vi "TB-Init History.vi"(0 "state":T1, 5 "Num Buffers":i32, 7 "XYGraph in":refnum<vi>) -> (4 "history":cluster{dbl[], dbl[]}[](array[cluster]))   [LabVIEW 2020]
uses:
  Typedefs/TB-Runtime state.ctl
  <vilib>/sound2/lvsound2.llb/Sound File Refnum.ctl
  Typedefs/TB-Setup Log.ctl
  Typedefs/TB-Analysis State.ctl
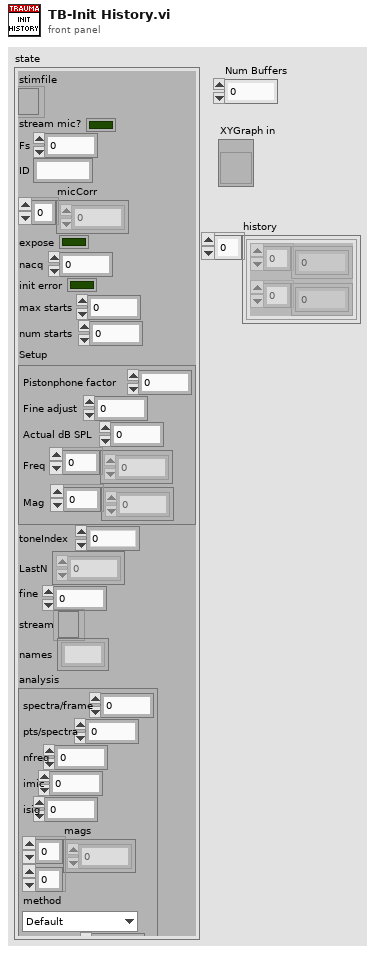
[diagram p1: front panel]
types:
  T1 = typedef "TB-Runtime state.ctl" = cluster{"stimfile":T2, "stream mic?":bool, "Fs":dbl, "ID":string, "micCorr":dbl[], "expose":bool, "nacq":i32, "init error":bool, "max starts":i32, "num starts":i32, "Setup":T3, "toneIndex":i32, "LastN":dbl[], "fine":dbl, "stream":refnum<file>, "names":string[], "analysis":T4}
  T2 = typedef "Sound File Refnum.ctl" = refnum<file>
  T3 = typedef "TB-Setup Log.ctl" = cluster{"Pistonphone factor":dbl, "Fine adjust":dbl, "Actual dB SPL":dbl, "Freq":dbl[], "Mag":dbl[]}
  T4 = typedef "TB-Analysis State.ctl" = cluster{"spectra/frame":i32, "pts/spectra":i32, "nfreq":i32, "imic":i32, "isig":i32, "mags":dbl[][], "method":enum16{"Default", "Periodogram", "Cross-spectrum"}, "cspd scale":dbl}
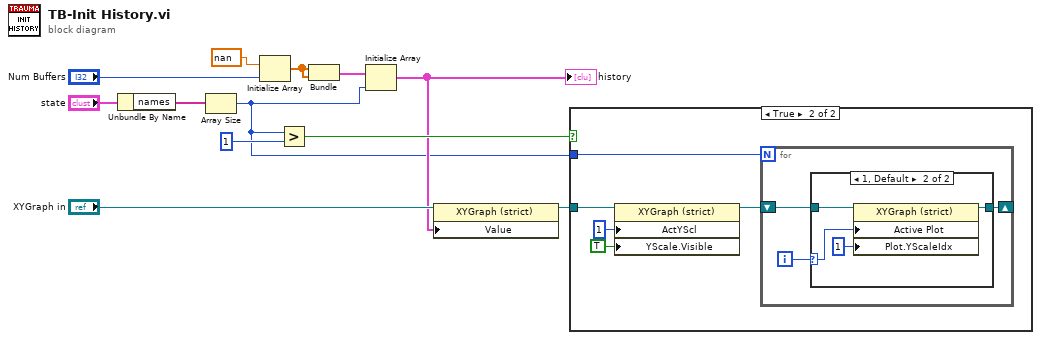
[diagram p0: block diagram]
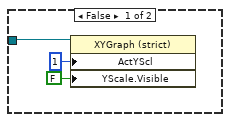
[diagram p2: hidden frame]
diagram:
  n1 = Unbundle By Name("state") -> ("names"=w11:string[])
  n2 = Array Size(array=w11) -> (size(s)=w1:i32)
  n3 = Initialize Array(nan ("element"), "Num Buffers") -> (w9:dbl[])
  n4 = Greater?(x=w1, y=1) -> (0:w6:bool)
  n5 = Bundle(w9, w9) -> (w8:cluster{dbl[], dbl[]})  [unwired: 1 in]
  n6 = Initialize Array(w8, w1) -> (w3:cluster{dbl[], dbl[]}[])
  "history" <- w3
  n7 = property class="XYGraph (strict)"(reference="XYGraph in", "Value"=w3) -> (reference out=w5:refnum<vi>)  [unwired: 1 in, 1 out]
  n8 = case shown="True" w6 {
    tunnel: w5 -> [w15 w18]
    tunnel: w1 -> [_ w16]
    frame False {
      n9 = property class="XYGraph (strict)"(reference=w15, "ActYScl"=1 ("Active Y Scale"), "YScale.Visible"=FALSE ("Y Scale.Visible")) -> ()  [unwired: 1 in, 2 out]
    }
    frame True {
      n10 = property class="XYGraph (strict)"(reference=w18, "ActYScl"=1 ("Active Y Scale"), "YScale.Visible"=TRUE ("Y Scale.Visible")) -> (reference out=w17:refnum<vi>)  [unwired: 1 in, 1 out]
      n11 = for {
        N: w16 -> [_]
        shift-right: [w22] -> _
        shift-left: w17 -> [w23]
        i -> [w21]
        n12 = case shown="1, Default" w21 {
          selector: w21 -> [_ w26]
          tunnel: w23 -> [w24 w28]
          tunnel: [w24 w27] -> w22
          frame 0 {
          }
          frame 1, Default {
            n13 = property class="XYGraph (strict)"(reference=w28, "Active Plot"=w26, "Plot.YScaleIdx"=u32 1 ("Plot.Y Scale Index")) -> (reference out=w27:refnum<vi>)  [unwired: 1 in, 1 out]
          }
        }
      }
    }
  }
